vi "Write Page.vi"(5 "byte order (0:big-endian, network order)":T4(ring), 6 "Settings":T1={"zlib compression level"=-1, "Max Strip bytes"=8192, "JPEG Quality (85)"=85}, 7 "Image Data":variant, 8 "error in (no error)":errorcluster, 9 "Details":T2 {"PhotometricInterpretation" items=["MIN IS WHITE"=0, "MIN IS BLACK"=1, "RGB"=2, "PALETTE"=3, "MASK"=4, "SEPARATED"=5, "YCBCR"=6, "CIE LAB"=8, "ICC LAB"=9, "ITU LAB"=10, "LOGL"=32844, "LOGLUV"=32845, "CFA"=32803, "LinearRaw"=34892, "DEPTH"=51177]}, 10 "Offset":i64, 11 "Byte Stream File in":refnum<file>) -> (0 "error out":errorcluster, 1 "IFD Baseline":T3 {"SampleFormat" items=["UINT"=1, "INT"=2, "FP"=3, "VOID"=4, "COMPLEXINT"=5, "COMPLEXFP"=6]; "NewSubFileType" items=["FILETYPE_REDUCEDIMAGE"=1, "FILETYPE_PAGE"=2, "FILETYPE_MASK"=4]; "Compression" items=["COMPRESSION_NONE"=1, "COMPRESSION_CCITTRLE"=2, "COMPRESSION_CCITTFAX3"=3, "COMPRESSION_CCITTFAX4"=4, "COMPRESSION_LZW"=5, "COMPRESSION_OJPEG"=6, "COMPRESSION_JPEG"=7, "COMPRESSION_NEXT"=32766, "COMPRESSION_CCITTRLEW"=32771, "COMPRESSION_PACKBITS"=32773, "COMPRESSION_THUNDERSCAN"=32809, "COMPRESSION_IT8CTPAD"=32895, "COMPRESSION_IT8LW"=32896, "COMPRESSION_IT8MP"=32897, "COMPRESSION_IT8BL"=32898, "COMPRESSION_PIXARFILM"=32908, "COMPRESSION_PIXARLOG"=32909, "COMPRESSION_DEFLATE"=32946, "COMPRESSION_ADOBE_DEFLATE"=8, "COMPRESSION_DSC"=32947, "COMPRESSION_JBIG"=34661, "COMPRESSION_SGILOG"=34676, "COMPRESSION_SGILOG24"=34677, "COMPRESSION_JP2000"=34712]; "PhotometricInterpretation" items=["PHOTOMETRIC_MINISWHITE"=0, "PHOTOMETRIC_MINISBLACK"=1, "PHOTOMETRIC_RGB"=2, "PHOTOMETRIC_PALETTE"=3, "PHOTOMETRIC_MASK"=4, "PHOTOMETRIC_SEPARATED"=5, "PHOTOMETRIC_YCBCR"=6, "PHOTOMETRIC_CIELAB"=8, "PHOTOMETRIC_ICCLAB"=9, "PHOTOMETRIC_ITULAB"=10, "PHOTOMETRIC_LOGL"=32844, "PHOTOMETRIC_LOGLUV"=32845, "CFA"=32803, "LinearRaw"=34892, "DEPTH"=51177]; "ResolutionUnit" items=["RESUNIT_NONE"=1, "RESUNIT_INCH"=2, "RESUNIT_CENTIMETER"=3]}, 2 "offset (in bytes)":i64, 3 "Byte Stream File out":refnum<file>)   [LabVIEW 2020, in "LV Tiff.lvlib"]
uses:
  LV Tiff.lvlib
  Baseline Tags 1.ctl
  Tiff Page Details.ctl
  Page Writer Settings.ctl
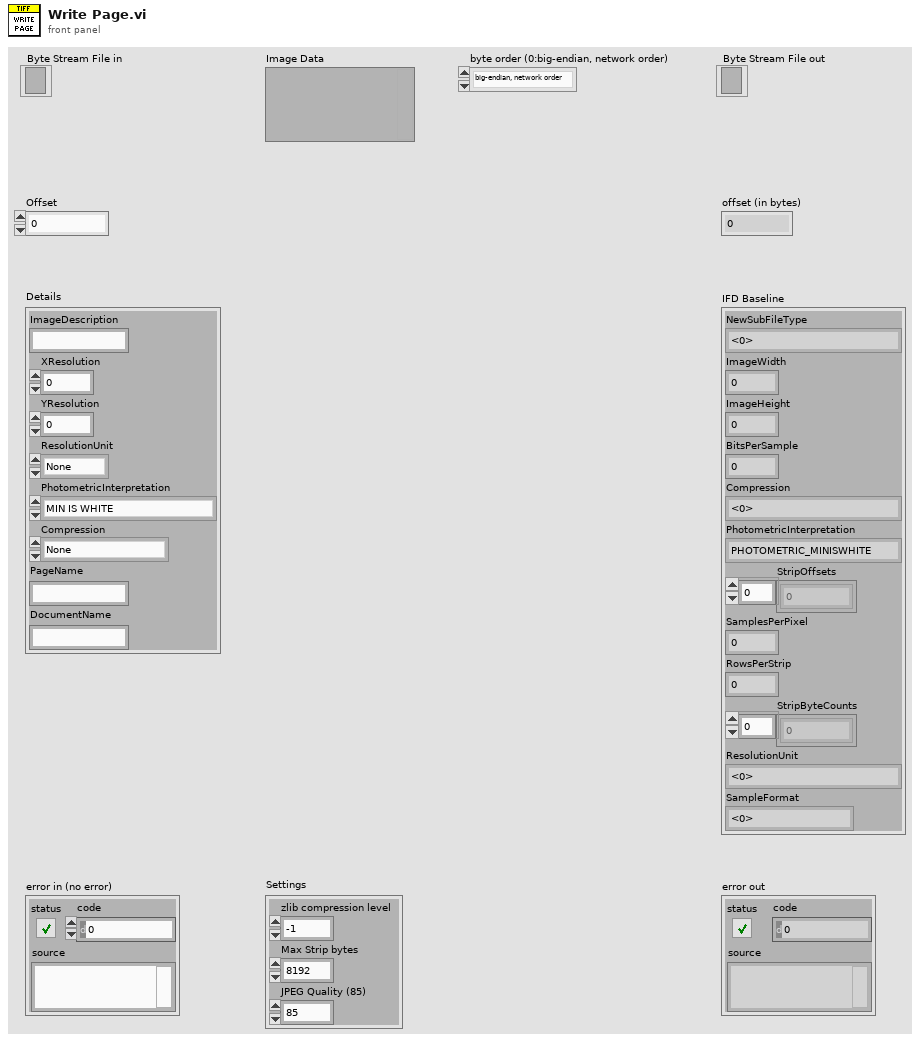
[diagram p1: front panel]
types:
  T1 = typedef "LV Tiff.lvlib/Page Writer Settings.ctl" = cluster{"zlib compression level":i32, "Max Strip bytes":u32, "JPEG Quality (85)":i32}
  T2 = typedef "LV Tiff.lvlib/Tiff Page Details.ctl" = cluster{"ImageDescription":string, "XResolution":dbl, "YResolution":dbl, "ResolutionUnit":enum16{"None", "Inch", "Centimeter"}, "PhotometricInterpretation":u16, "Compression":enum16{"None", "Deflate", "JPEG"}, "PageName":string, "DocumentName":string}
  T3 = typedef "LV Tiff.lvlib/Baseline Tags 1.ctl" = cluster{"NewSubFileType":u32, "ImageWidth":u32, "ImageHeight":u32, "BitsPerSample":u16, "Compression":u16, "PhotometricInterpretation":u16, "StripOffsets":u32[], "SamplesPerPixel":u16, "RowsPerStrip":u32, "StripByteCounts":u32[], "ResolutionUnit":u16, "SampleFormat":u16}
  T4 = enum16{"big-endian, network order", "native, host order", "little-endian"}
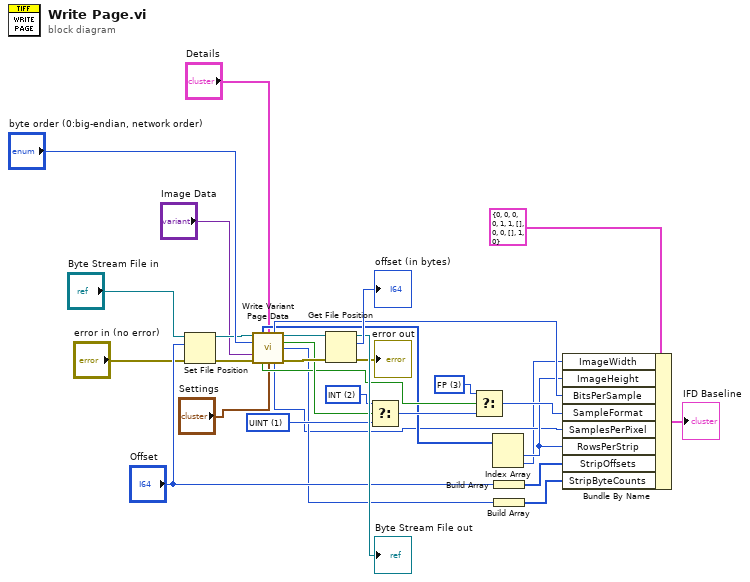
[diagram p0: block diagram]
diagram:
  w23 = u16 3 items=["UINT"=1, "INT"=2, "FP"=3, "VOID"=4, "COMPLEXINT"=5, "COMPLEXFP"=6] ("SampleFormat")
  w25 = u16 2 items=["UINT"=1, "INT"=2, "FP"=3, "VOID"=4, "COMPLEXINT"=5, "COMPLEXFP"=6] ("SampleFormat")
  w26 = u16 1 items=["UINT"=1, "INT"=2, "FP"=3, "VOID"=4, "COMPLEXINT"=5, "COMPLEXFP"=6] ("SampleFormat")
  n1 = Set File Position(offset (in bytes) (0)="Offset", refnum="Byte Stream File in", error in="error in (no error)") -> (refnum out=w20:refnum<file>, error out=w9:errorcluster)  [unwired: 1 in]
  n2 = call "Write Variant Page Data.vi"("Byte Stream File in"=w20, "Details"="Details", "byte order (0:big-endian, network order)"="byte order (0:big-endian, network order)", "Image Data"="Image Data", "error in (no error)"=w9, "Settings"="Settings") -> ("Size(s)"=w12:u32[], "Bits per Sample"=w13:u32, "Byte Stream File out"=w17:refnum<file>, "Signed"=w15:bool, "Data Bytes"=w7:i64, "Fractional"=w14:bool, "Samples Per Pixel"=w5:i32, "error out"=w18:errorcluster)  [unwired: 1 in, 1 out]
  n3 = Get File Position(4:w18, 7:w17) -> (0:→"error out":errorcluster, 2:→"offset (in bytes)":i64, 3:→"Byte Stream File out":refnum<file>)
  n4 = Select(t=w25, s=w15, f=w26) -> (s? t:f=w24:u16)
  n5 = Select(t=w23, s=w14, f=w24) -> (s? t:f=w22:u16)
  n6 = Index Array(array=w12) -> (element #1=w6:u32, element #2=w4:u32)  [unwired: 2 in]
  n7 = Build Array("Offset") -> (w2:i64[])
  n8 = Build Array(w7) -> (w3:i64[])
  n9 = Bundle By Name(cluster=T3 {"NewSubFileType"=0, "ImageWidth"=0, "ImageHeight"=0, "BitsPerSample"=0, "Compression"=1, "PhotometricInterpretation"=1, "StripOffsets"=[], "SamplesPerPixel"=0, "RowsPerStrip"=0, "StripByteCounts"=[], "ResolutionUnit"=1, "SampleFormat"=0} ("Cluster"), "ImageWidth"=w4, "ImageHeight"=w6, "BitsPerSample"=w13, "SampleFormat"=w22, "SamplesPerPixel"=w5, "RowsPerStrip"=w6, "StripOffsets"=w2, "StripByteCounts"=w3) -> (→"IFD Baseline":T3)
